vi "Increasing Count.vi"() -> ()   [LabVIEW 2020]
uses:
  <vilib>/regexp/Match Regular Expression.xnode
panel:
  out "Increasing Count":i32
  in  "Input":string="156\n153\n163\n168\n166\n164\n149\n187\n192\n194\n197\n199\n201\n210\n211\n196\n202\n203\n193\n199\n236\n240\n241\n251\n228\n226\n227\n256\n269\n270\n265\n271\n267\n271\n247\n254\n259\n258\n269\n270\n269\n267\n289\n290\n288\n309\n307\n299\n309\n326\n329\n332\n335\n338\n342\n333\n330\n332\n333\n334\n318\n317\n318\n316\n314\n315\n322\n327\n328\n331\n332\n338\n346\n341\n350\n334\n323\n322\n321\n325\n329\n342\n343\n353\n361\n355\n331\n329\n330\n319\n321\n322\n321\n322\n325\n316\n317\n322\n324\n331\n322\n323\n324\n325\n324\n336\n324\n335\n336\n337\n335\n336\n339\n343\n348\n353\n351\n349\n339\n341\n327\n322\n325\n298\n299\n306\n307\n321\n317\n314\n313\n316\n328\n325\n330\n331\n332\n339\n340\n348\n352\n354\n350\n374\n364\n370\n371\n379\n381\n380\n..."
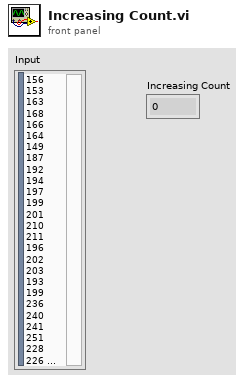
[diagram p1: front panel]
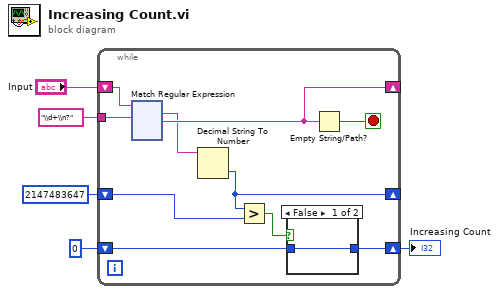
[diagram p0: block diagram]
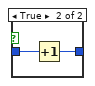
[diagram p2: hidden frame]
diagram:
  n1 = while {
    shift-right: [w13] -> _
    shift-left: "Input" -> [w6]
    tunnel: "\\d+\\n?" -> [w15]
    shift-right: [w12] -> _
    shift-left: 2147483647 -> [w11]
    shift-right: [w8] -> w1
    shift-left: 0 -> [w9]
    stop <- w14 stop-if-true
    n2 = xnode "Match Regular Expression"("input string"=w6, "regular expression"=w15) -> ("whole match"=w7:string, "after match"=w13:string)  [unwired: 4 in, 3 out]
    n3 = Decimal String To Number(string=w7) -> (number=w12:i32)  [unwired: 2 in, 1 out]
    n4 = Greater?(x=w12, y=w11) -> (0:w10:bool)
    n5 = case shown="False" w10 {
      tunnel: w9 -> [w130 w132]
      tunnel: [w130 w131] -> w8
      frame False {
      }
      frame True {
        n6 = Increment(x=w132) -> (x+1=w131:i32)
      }
    }
    n7 = Empty String/Path?(string/path=w13) -> (empty?=w14:bool)
  }
  "Increasing Count" <- w1
